vi "setTemperature.vi"(6 "Channel":i32, 8 "error in (no error)":errorcluster, 9 "Rate (K/min)":dbl, 10 "Temperature (K)":dbl, 11 "Instrument.Cryostat in":refnum<class "Instrument.Cryostat.lvclass">) -> (0 "error out":errorcluster, 3 "Instrument.Cryostat out":refnum<class "Instrument.Cryostat.lvclass">)   [LabVIEW 2019, in "Instrument.Cryostat.lvclass"]
uses:
  Instrument.Cryostat.lvclass
  Typedefs/setTemperature--cluster.ctl
  Typedefs/Cryostat.commands--enum.ctl
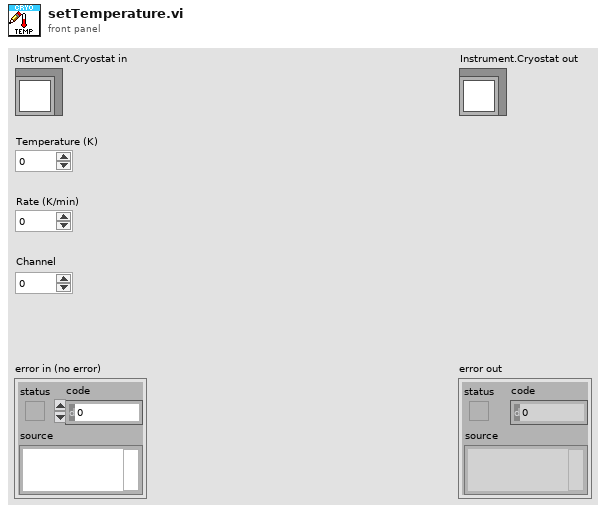
[diagram p1: front panel]
types:
  T1 = typedef "Instrument.Cryostat.lvclass/Cryostat.commands--enum.ctl" = enum16{"getLN2Level", "getLHeLevel", "getMagnet", "getMagnetVector", "setMagnet", "setMagnetVector", "getAngle", "setAngle", "getTemperature", "setTemperature", "getHeater", "setHeater", "getChamber", "setChamber", "getPressure"}
  T2 = typedef "Instrument.Cryostat.lvclass/setTemperature--cluster.ctl" = cluster{"temperature":dbl, "rate":dbl, "channel":i32}
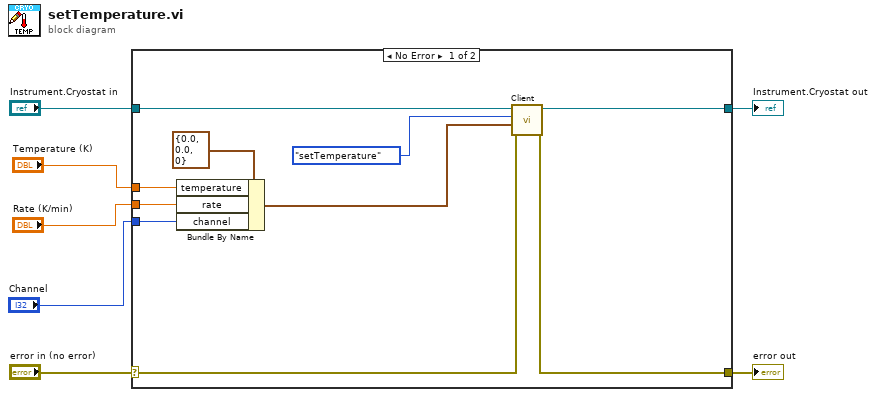
[diagram p0: block diagram]
diagram:
  n1 = case shown="No Error" "error in (no error)" {
    selector: "error in (no error)" -> [w9 w19]
    tunnel: [w11 w19] -> w6
    tunnel: [w12 w18] -> w4
    tunnel: "Instrument.Cryostat in" -> [w10 w18]
    tunnel: "Temperature (K)" -> [w16 _]
    tunnel: "Rate (K/min)" -> [w15 _]
    tunnel: "Channel" -> [w14 _]
    frame No Error {
      n2 = Bundle By Name(cluster=T2 {"temperature"=0.0, "rate"=0.0, "channel"=0} ("Set Temperature"), "temperature"=w16, "rate"=w15, "channel"=w14) -> (w13:T2)
      n3 = call-dynamic "Client.vi"("error in (no error)"=w9, "Data in"=w13, "Command in"=Cryostat.commands--enum."setTemperature" ("commands"), "Instrument in"=w10) -> ("error out"=w11:errorcluster, "Instrument out"=w12:refnum<class "Instrument.Cryostat.lvclass">)  [unwired: 4 in, 2 out]
    }
    frame Error {
    }
  }
  "error out" <- w6
  "Instrument.Cryostat out" <- w4
